vi "CRYCalc Res Standard deviation.vi"(6 "Statistic Run Number":i32, 7 "Step Setup VI No":i32, 8 "Work in":u16, 9 "+/-Adjust(Deviation)":i32, 11 "Results in":T2 {"Margin" format="%.2f"}) -> (1 "Margin Std Dev Out":T1[](array[typedef]) {"Z data" items=["dB", "Lin"]; "X data" items=["dB", "Lin"]; "Y data" items=["dB", "Lin"]; "Z dB ref" format="%.1f"; "Z axis" items=["Log", "Lin"]; "X dB ref" format="%.1f"; "X axis" items=["Log", "Lin"]; "Y axis" items=["Log", "Lin"]; "Y dB ref" format="%.1f"; "Curve"."z" format="%.2f"; "Curve"."y" format="%.2f"; "Curve"."x" format="%.2f"}, 2 "Margin mean Out":T1[](array[typedef]) {"Z data" items=["dB", "Lin"]; "X data" items=["dB", "Lin"]; "Y data" items=["dB", "Lin"]; "Z dB ref" format="%.1f"; "Z axis" items=["Log", "Lin"]; "X dB ref" format="%.1f"; "X axis" items=["Log", "Lin"]; "Y axis" items=["Log", "Lin"]; "Y dB ref" format="%.1f"; "Curve"."z" format="%.2f"; "Curve"."y" format="%.2f"; "Curve"."x" format="%.2f"}, 3 "Standard Dev Out":T1[](array[typedef]) {"Z data" items=["dB", "Lin"]; "X data" items=["dB", "Lin"]; "Y data" items=["dB", "Lin"]; "Z dB ref" format="%.1f"; "Z axis" items=["Log", "Lin"]; "X dB ref" format="%.1f"; "X axis" items=["Log", "Lin"]; "Y axis" items=["Log", "Lin"]; "Y dB ref" format="%.1f"; "Curve"."z" format="%.2f"; "Curve"."y" format="%.2f"; "Curve"."x" format="%.2f"})   [LabVIEW 2013]
uses:
  Typedef Control/CRYResult Cluster Array.ctl
  Typedef Control/CRYResult Cluster.ctl
  Typedef Control/CRYData Cluster.ctl
  Typedef Control/CRYData Cluster Array.ctl
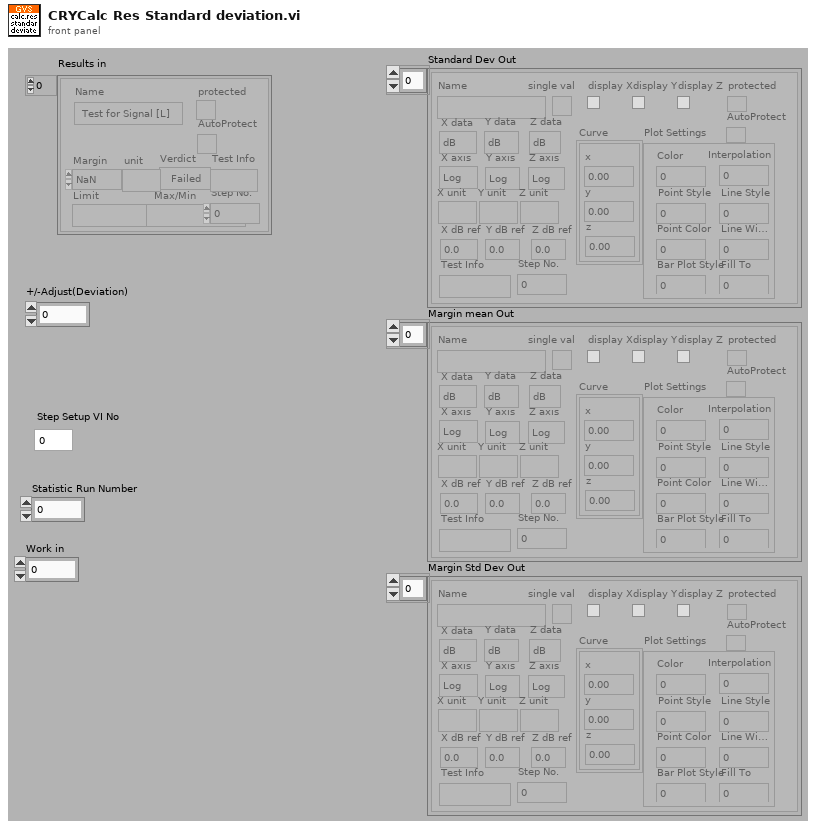
[diagram p1: front panel]
types:
  T1 = typedef "CRYData Cluster.ctl" = cluster{"Name":string, "Curve":cluster{"x":dbl, "y":dbl, "z":dbl}[], "X data":u16, "Y data":u16, "Z data":u16, "X axis":u16, "Y axis":u16, "Z axis":u16, "X unit":string, "Y unit":string, "Z unit":string, "X dB ref":dbl, "Y dB ref":dbl, "Z dB ref":dbl, "single val":bool, "protected":bool, "display X":bool, "display Y":bool, "display Z":bool, "Test Info":string, "Step No.":i32, "Plot Settings":cluster{"Color":u32, "Interpolation":u8, "Point Style":u8, "Line Style":u8, "Point Color":u32, "Line Width":u8, "Bar Plot Style":u8, "Fill To":i16}, "AutoProtect":bool}
  T2 = typedef "CRYResult Cluster Array.ctl" = T3[]
  T3 = typedef "CRYResult Cluster.ctl" = cluster{"Name":string, "Margin":dbl, "unit":string, "Verdict":bool, "Limit":string, "Max/Min":string, "protected":bool, "Step No.":i32, "Test Info":string, "AutoProtect":bool}
  T4 = typedef "CRYData Cluster Array.ctl" = T1[]
  T5 = enum32{"English", "Chinese", "Korean", "Japanese", "Russian", "Chinese traditional"}
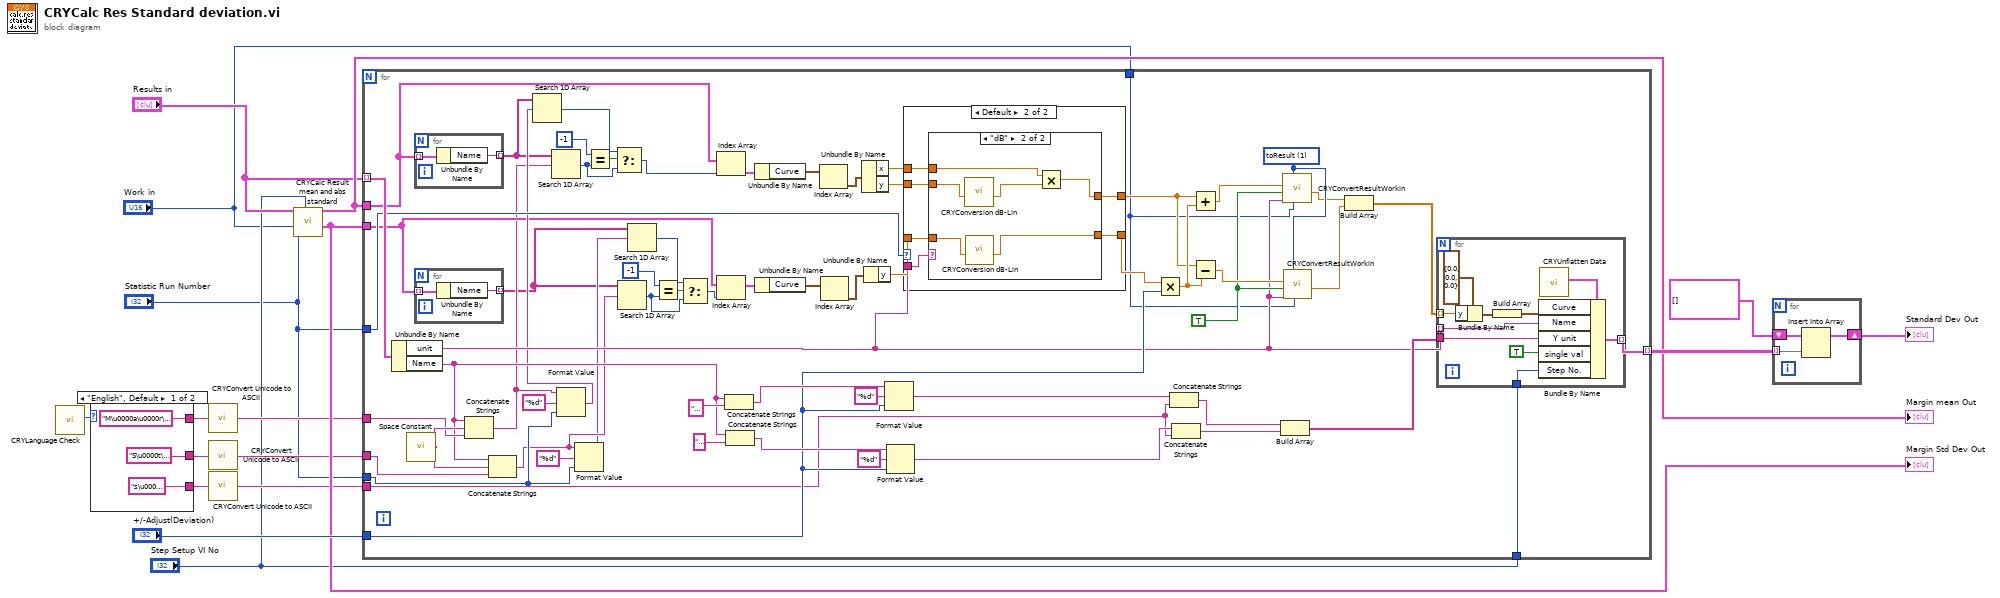
[diagram p0: block diagram]
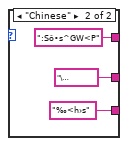
[diagram p2: hidden frame]
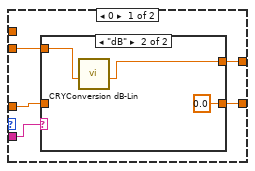
[diagram p3: hidden frame]
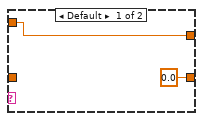
[diagram p4: hidden frame]
diagram:
  n1 = call "CRYLanguage Check.vi"() -> ("Language"=w9:T5)  [unwired: 10 in, 1 out]
  n2 = case shown="\"English\", Default" w9 {
    tunnel: ["M\u0000a\u0000r\u0000g\u0000i\u0000n\u0000 \u0000M\u0000e\u0000a\u0000n\u0000" ("format string") ":Sô•s^GW<P" ("format string")] -> w10
    tunnel: ["S\u0000t\u0000d\u0000 \u0000D\u0000e\u0000v\u0000" ("format string") "\u0007hÆQî]" ("format string")] -> w8
    tunnel: ["s\u0000i\u0000g\u0000m\u0000a\u0000" ("format string") "‰<h›s" ("format string")] -> w5
    frame "English", Default {
    }
    frame "Chinese" {
    }
  }
  n3 = call "CRYConvert Unicode to ASCII.vi"("Unicode"=w10) -> ("ASCII"=w7:string)  [unwired: 4 in]
  n4 = call "CRYConvert Unicode to ASCII.vi"("Unicode"=w8) -> ("ASCII"=w6:string)  [unwired: 4 in]
  n5 = call "CRYConvert Unicode to ASCII.vi"("Unicode"=w5) -> ("ASCII"=w4:string)  [unwired: 4 in]
  n6 = call "CRYCalc Result mean and abs standard.vi"("Step Setup VI No"="Step Setup VI No", "Statistic Run Number"="Statistic Run Number", "Work in"="Work in", "Results in"="Results in") -> ("Margin Std Dev Out"=w12:T1[], "Margin mean Out"=w13:T1[])  [unwired: 5 in, 1 out]
  "Margin mean Out" <- w13
  "Margin Std Dev Out" <- w12
  n7 = for {
    tunnel: "+/-Adjust(Deviation)" -> [w64]
    tunnel: "Results in" -> [w60] mode=indexing
    tunnel: [w85] -> w15 mode=indexing
    tunnel: w13 -> [w37]
    tunnel: w12 -> [w40]
    tunnel: "Step Setup VI No" -> [w77]
    tunnel: w7 -> [w76]
    tunnel: w6 -> [w75]
    tunnel: w4 -> [w63]
    tunnel: "Statistic Run Number" -> [w59]
    tunnel: "Work in" -> [w49]
    tunnel: "Statistic Run Number" -> [w41]
    w51 = TRUE ("IsTrue")
    w52 = u16 1 items=["toWorkin", "toResult"] ("Type")
    n8 = Unbundle By Name(w60) -> ("unit"=w50:string, "Name"=w62:string)
    n9 = call <vilib>:"Space Constant.vi"() -> ("String"=w84:string)
    n10 = for {
      tunnel: w37 -> [w88] mode=indexing
      tunnel: [w87] -> w33 mode=indexing
      n11 = Unbundle By Name(w88) -> ("Name"=w87:string)
    }
    n12 = for {
      tunnel: w40 -> [w90] mode=indexing
      tunnel: [w89] -> w27 mode=indexing
      n13 = Unbundle By Name(w90) -> ("Name"=w89:string)
    }
    n14 = Concatenate Strings(w62, w84, w76) -> (w34:string)
    n15 = Concatenate Strings(w62, w84, w75) -> (w29:string)
    n16 = Search 1D Array(1D array=w33, element=w34) -> (index of element=w31:i32)  [unwired: 1 in]
    n17 = Format Value(string ("")=w34, format string="%d", value (0)=w41) -> (output string=w43:string)
    n18 = Search 1D Array(1D array=w33, element=w43) -> (index of element=w32:i32)  [unwired: 1 in]
    n19 = Format Value(string ("")=w29, format string="%d", value (0)=w41) -> (output string=w28:string)
    n20 = Equal?(x=-1, y=w31) -> (x = y?=w35:bool)
    n21 = Select(t=w32, s=w35, f=w31) -> (s? t:f=w30:i32)
    n22 = Search 1D Array(1D array=w27, element=w29) -> (index of element=w25:i32)  [unwired: 1 in]
    n23 = Search 1D Array(1D array=w27, element=w28) -> (index of element=w26:i32)  [unwired: 1 in]
    n24 = Equal?(x=-1, y=w25) -> (x = y?=w39:bool)
    n25 = Select(t=w26, s=w39, f=w25) -> (s? t:f=w24:i32)
    n26 = Index Array(array=w37, index=w30) -> (element=w83:T1)
    n27 = Index Array(array=w40, index=w24) -> (element=w82:T1)
    n28 = Concatenate Strings(w62, "+\u0000" ("format string")) -> (w73:string)
    n29 = Concatenate Strings(w62, "-\u0000" ("format string")) -> (w74:string)
    n30 = Unbundle By Name(w83) -> ("Curve"=w81:cluster{"x":dbl, "y":dbl, "z":dbl}[])
    n31 = Unbundle By Name(w82) -> ("Curve"=w80:cluster{"x":dbl, "y":dbl, "z":dbl}[])
    n32 = Index Array(array=w81) -> (element=w79:cluster{"x":dbl, "y":dbl, "z":dbl})  [unwired: 1 in]
    n33 = Index Array(array=w80) -> (element=w78:cluster{"x":dbl, "y":dbl, "z":dbl})  [unwired: 1 in]
    n34 = Unbundle By Name(w79) -> ("x"=w45:dbl, "y"=w58:dbl)
    n35 = Unbundle By Name(w78) -> ("y"=w57:dbl)
    n36 = Format Value(string ("")=w73, format string="%d", value (0)=w64) -> (output string=w69:string)
    n37 = Format Value(string ("")=w74, format string="%d", value (0)=w64) -> (output string=w70:string)
    n38 = case shown="Default" w59 {
      tunnel: w58 -> [w95 w105]
      tunnel: w57 -> [w94 w102]
      tunnel: w50 -> [w91 w106]
      tunnel: [w92 w104] -> w56
      tunnel: [w93 w103] -> w55
      tunnel: w45 -> [_ w101]
      frame 0 {
        n39 = case shown="\"dB\"" w91 {
          tunnel: w95 -> [w97 w100]
          tunnel: [w97 w99] -> w92
          tunnel: [0.0 0.0] -> w93
          tunnel: w94 -> [_ _]
          frame Default {
          }
          frame "dB" {
            n40 = call "CRYConversion dB-Lin.vi"("Log In"=w100) -> ("Lin Out"=w99:dbl)  [unwired: 5 in, 3 out]
          }
        }
      }
      frame Default {
        n41 = case shown="\"dB\"" w106 {
          tunnel: w105 -> [w108 w114]
          tunnel: [w108 w110] -> w104
          tunnel: [w107 w109] -> w103
          tunnel: w102 -> [w107 w113]
          tunnel: w101 -> [_ w111]
          frame Default {
          }
          frame "dB" {
            n42 = call "CRYConversion dB-Lin.vi"("Log In"=w114) -> ("Lin Out"=w112:dbl)  [unwired: 5 in, 3 out]
            n43 = call "CRYConversion dB-Lin.vi"("Log In"=w113) -> ("Lin Out"=w109:dbl)  [unwired: 5 in, 3 out]
            n44 = Multiply(x=w111, y=w112) -> (x*y=w110:dbl)
          }
        }
      }
    }
    n45 = Multiply(x=w55, y=w64) -> (x*y=w86:dbl)
    n46 = Concatenate Strings(w69, w63) -> (w71:string)
    n47 = Concatenate Strings(w70, w63) -> (w72:string)
    n48 = Add(x=w56, y=w86) -> (x+y=w53:dbl)
    n49 = Subtract(x=w56, y=w86) -> (x-y=w54:dbl)
    n50 = Build Array(w71, w72) -> (w61:string[])
    n51 = call "CRYConvertResultWorkin.vi"("Work in"=w49, "Type"=w52, "unit"=w50, "IsTrue"=w51, "Margin In"=w53) -> ("Margin Out"=w48:dbl)  [unwired: 6 in]
    n52 = call "CRYConvertResultWorkin.vi"("Work in"=w49, "Type"=w52, "unit"=w50, "IsTrue"=w51, "Margin In"=w54) -> ("Margin Out"=w47:dbl)  [unwired: 6 in]
    n53 = Build Array(w48, w47) -> (w46:dbl[])
    n54 = for {
      tunnel: w61 -> [w120] mode=indexing
      tunnel: [w119] -> w85 mode=indexing
      tunnel: w46 -> [w118] mode=indexing
      tunnel: w77 -> [w117]
      tunnel: w50 -> [w115]
      n55 = Bundle By Name(cluster=cluster{"x":dbl, "y":dbl, "z":dbl} {"x"=0.0, "y"=0.0, "z"=0.0}, "y"=w118) -> (w124:cluster{"x":dbl, "y":dbl, "z":dbl})
      n56 = Build Array(w124) -> (w121:cluster{"x":dbl, "y":dbl, "z":dbl}[])
      n57 = call "CRYUnflatten Data.vi"() -> ("Datum"=w116:T1)  [unwired: 9 in, 2 out]
      n58 = Bundle By Name(cluster=w116, "Curve"=w121, "Name"=w120, "Y unit"=w115, "single val"=TRUE, "Step No."=w117) -> (w119:T1)
    }
  }
  n59 = for {
    tunnel: w15 -> [w127] mode=indexing
    shift-right: [w125] -> w14
    shift-left: T4 [] ("Data in") -> [w126]
    n60 = Insert Into Array(array=w126, new element=w127) -> (w125:T4)  [unwired: 1 in]
  }
  "Standard Dev Out" <- w14
